vi "Check CSV Error.vi"(8 "error in (no error)":errorcluster) -> (0 "error out":errorcluster)   [LabVIEW 2025, in "I2C Bus Monitor UI.lvlib"]
uses:
  I2C Bus Monitor UI.lvlib
  Save CSV.vi
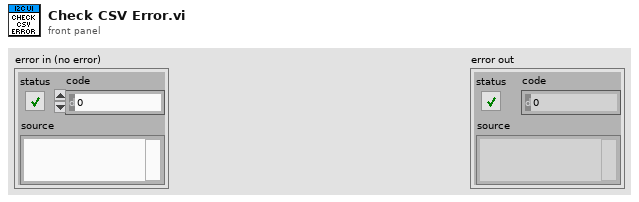
[diagram p1: front panel]
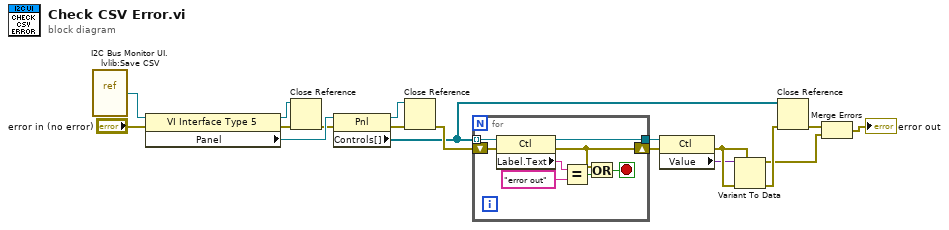
[diagram p0: block diagram]
diagram:
  n1 = vi-ref "I2C Bus Monitor UI.lvlib:Save CSV.vi"() -> (w17:refnum<vi>)
  n2 = property class="VI Interface Type 5"(reference=w17, error in="error in (no error)") -> (reference out=w9:refnum<vi>, error out=w14:errorcluster, "Panel"=w15:refnum<vi>)
  n3 = Close Reference(reference=w9, error in (no error)=w14) -> (error out=w10:errorcluster)
  n4 = property class="Pnl"(reference=w15, error in=w10) -> (reference out=w7:refnum<vi>, error out=w13:errorcluster, "Controls[]"=w5:refnum<vi>[])
  n5 = Close Reference(reference=w7, error in (no error)=w13) -> (error out=w8:errorcluster)
  n6 = for {
    tunnel: w5 -> [w26] mode=indexing
    tunnel: [w23] -> w11
    shift-right: [w19] -> w12
    shift-left: w8 -> [w21]
    stop <- w20 stop-if-true
    n7 = property class="Ctl"(reference=w26, error in=w21) -> (reference out=w23:refnum<vi>, error out=w19:errorcluster, "Label.Text"=w25:string)
    n8 = Equal?(x=w25, y="error out" ("Label.Text")) -> (x = y?=w22:bool)
    n9 = Or(x=w19, y=w22) -> (x .or. y?=w20:bool)
  }
  n10 = property class="Ctl"(reference=w11, error in=w12) -> (error out=w18:errorcluster, "Value"=w3:variant)  [unwired: 1 out]
  n11 = Variant To Data(error in=w18, type=w18, Variant=w3) -> (data=w1:errorcluster, error out=w2:errorcluster)
  n12 = Close Reference(reference=w5, error in (no error)=w2) -> (error out=w6:errorcluster)
  n13 = Merge Errors(w6, w1) -> (→"error out":errorcluster)
